vi "Send ILC Outputs.vi"(8 "error in (no error)":errorcluster, 11 "Model in":refnum<class "Model.lvclass">) -> (0 "error out":errorcluster, 3 "Model out":refnum<class "Model.lvclass">)   [LabVIEW 2015, in "Model.lvclass"]
uses:
  Model.lvclass
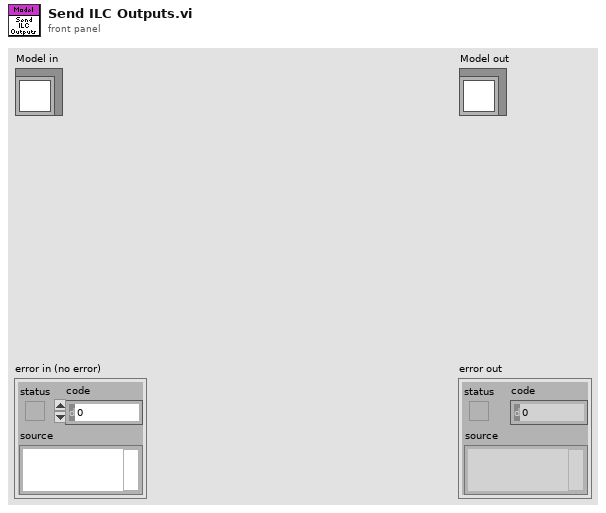
[diagram p1: front panel]
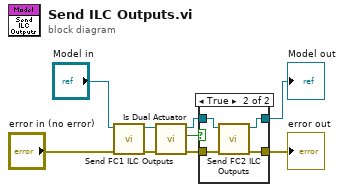
[diagram p0: block diagram]
diagram:
  n1 = call "Send FC1 ILC Outputs.vi"("error in (no error)"="error in (no error)", "Model in"="Model in") -> ("error out"=w2:errorcluster, "Model out"=w1:refnum<class "Model.lvclass">)  [unwired: 8 in]
  n2 = call "Is Dual Actuator.vi"("error in (no error)"=w2, "Model in"=w1) -> ("error out"=w3:errorcluster, "Is Dual Actuator"=w7:bool, "Model out"=w6:refnum<class "Model.lvclass">)  [unwired: 7 in]
  n3 = case shown="True" w7 {
    tunnel: w6 -> [w11 w15]
    tunnel: [w11 w14] -> w5
    tunnel: [w10 w13] -> w4
    tunnel: w3 -> [w10 w12]
    frame False {
    }
    frame True {
      n4 = call "Send FC2 ILC Outputs.vi"("error in (no error)"=w12, "Model in"=w15) -> ("error out"=w13:errorcluster, "Model out"=w14:refnum<class "Model.lvclass">)  [unwired: 8 in]
    }
  }
  "error out" <- w4
  "Model out" <- w5
